vi "pkpk_rms_subvi.vi"(11 "Array":dbl[](array[numeric])) -> (2 "RMS":dbl, 3 "Pk-Pk":dbl)   [LabVIEW 2020]
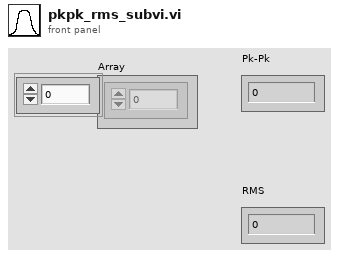
[diagram p1: front panel]
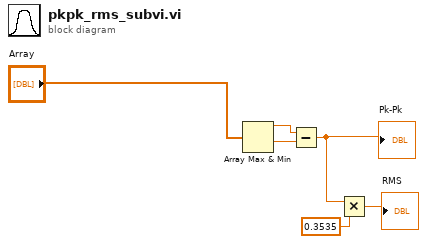
[diagram p0: block diagram]
diagram:
  n1 = Array Max & Min(array="Array") -> (max value=w1:dbl, min value=w4:dbl)  [unwired: 2 out]
  n2 = Subtract(x=w1, y=w4) -> (x-y=w3:dbl)
  "Pk-Pk" <- w3
  n3 = Multiply(x=w3, y=0.3535) -> (x*y=→"RMS":dbl)
